vi "StartProgram.vi"() -> ()   [LabVIEW 2018]
uses:
  Type_Def/TypeDef_BMSData.ctl
  Type_Def/TypeDef_BmsStatus.ctl
  Type_Def/TypeDef_cRIOData.ctl
  Master/TypeDef_LoopPeriods.ctl
  <vilib>/Utility/error.llb/Error Cluster From Error Code.vi
  <vilib>/rvi/errors/niLvFpgaAdjustHostInterfaceError.vi
  <vilib>/rvi/interface/nirviReadWriteControl/nirviReadWriteControl.xnode
  <vilib>/NI_Real-Time Target Support.lvlib
  NiFpgaLv.dll
  <vilib>/rvi/interface/Simulation/niFpgaSimulationCallBeginRW.vi
panel:
  in  "error in (no error)":errorcluster
  out "FPGA VI Reference In 2":refnum<k20>
  in  "FPGA VI Reference In":refnum<k20>
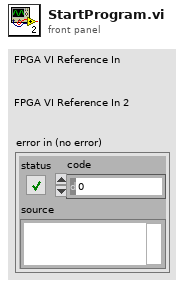
[diagram p1: front panel]
types:
  T1 = typedef "TypeDef_cRIOData.ctl" = cluster{"Time (ms)":dbl, "24V Battery (V)":dbl, "LowV Current (A)":dbl, "Fiducial Sensor (V)":dbl, "PV Pressure (psig)":dbl, "Flow Sensor (V)":dbl, "Temp Fairing (F)":dbl, "Temp Reservoir (F)":dbl, "HallEffect Right (in)":dbl, "HallEffect Left (in)":dbl, "PT Tank (psig)":dbl, "PT Clamp Right (psig)":dbl, "PT Clamp Left (psig)":dbl, "PT Brake (psig)":dbl, "PT Cooling (psig)":dbl, "Displacement (ft)":dbl, "Velocity (ft/s)":dbl}
  T2 = typedef "TypeDef_BMSData.ctl" = cluster{"Max Cell Voltage (V)":dbl, "Max Cell ID":dbl, "Min Cell Voltage (V)":dbl, "Min Cell ID":dbl, "State of Charge (%)":dbl, "Average Voltage (V)":dbl, "Voltage Delta (V)":dbl, "Pack Current (A)":dbl, "Pack Voltage (V)":dbl, "Max Resistance (Ohm)":dbl, "Min Resistance (Ohm)":dbl, "Average Resistance (Ohm)":dbl, "Delta Resistance (Ohm)":dbl, "Highest Temperature(F)":dbl, "BmsStatus":T3}
  T3 = typedef "TypeDef_BmsStatus.ctl" = cluster{"isFault":bool, "isolationMonitoring":bool}
  T4 = typedef "TypeDef_LoopPeriods.ctl" = cluster{"Control Period":i64, "DAQ Period":u32, "IMU Period":u32, "CAN Period":i64, "Nav Period":u32}
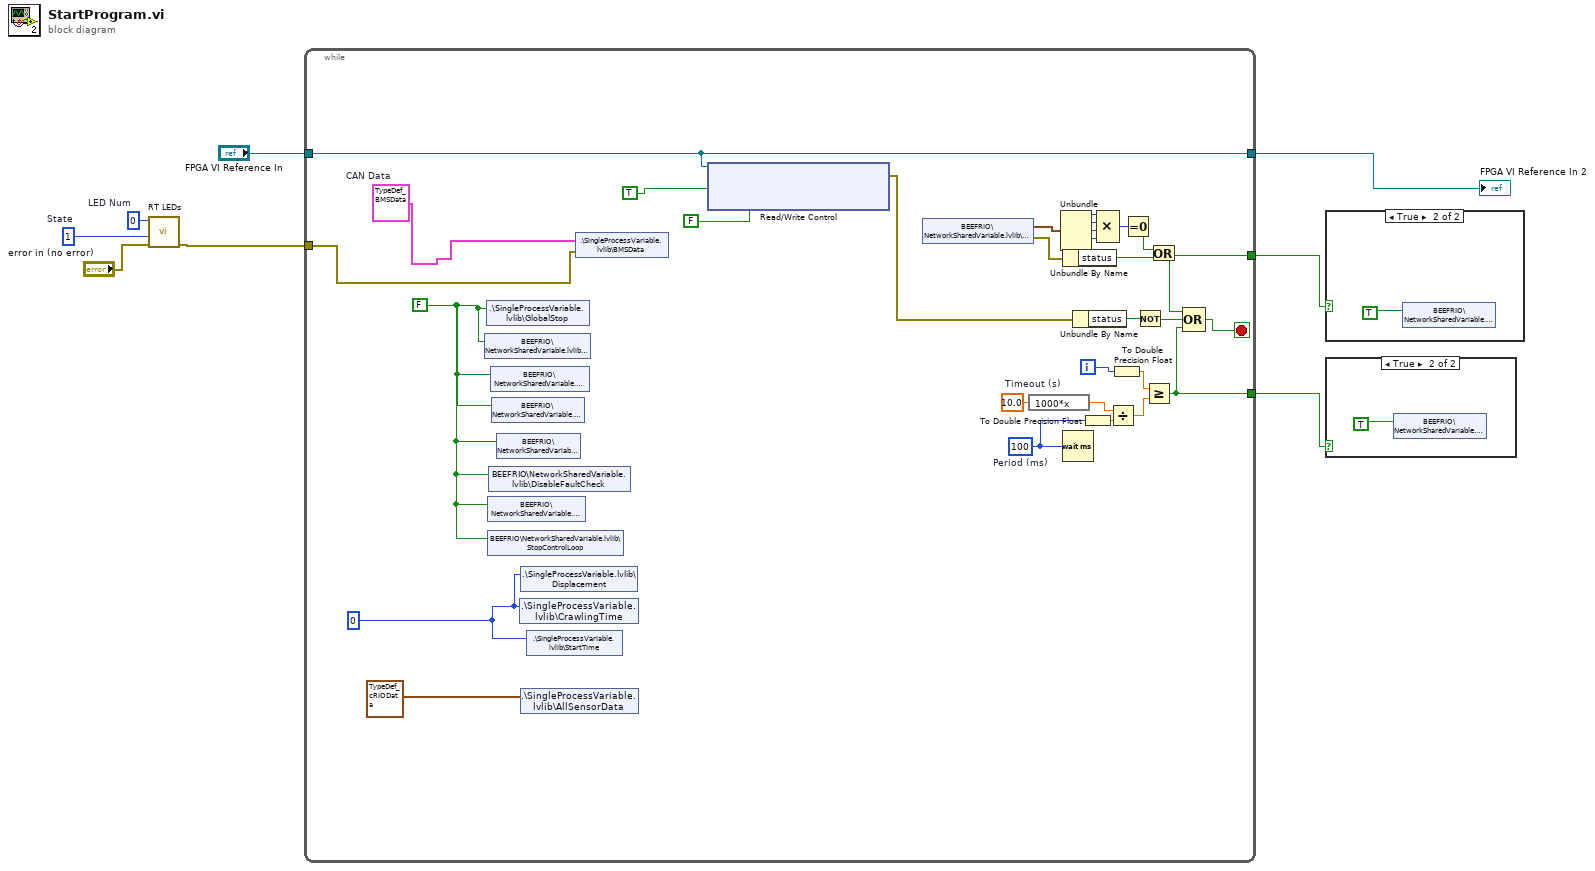
[diagram p0: block diagram]
diagram:
  w5 = 1  # State
  w6 = 0  # LED Num
  n1 = call <vilib>:"RT LEDs.vi"("error in (no error)"="error in (no error)", "State"=w5, "LED Num"=w6) -> ("error out"=w3:errorcluster)  [unwired: 3 in, 1 out]
  n2 = while {
    tunnel: [w32] -> w8
    tunnel: "FPGA VI Reference In" -> [w32]
    tunnel: w3 -> [w37]
    tunnel: [w12] -> w2
    tunnel: [w11] -> w1
    i -> [w9]
    stop <- w13 stop-if-true
    w29 = 10.0  # Timeout (s)
    w27 = u32 100  # Period (ms)
    w36 = i64 0 ("StartTime")
    w35 = FALSE ("GlobalStop")
    w38 = T2 {"Max Cell Voltage (V)"=0.0, "Max Cell ID"=0.0, "Min Cell Voltage (V)"=0.0, "Min Cell ID"=0.0, "State of Charge (%)"=0.0, "Average Voltage (V)"=0.0, "Voltage Delta (V)"=0.0, "Pack Current (A)"=0.0, "Pack Voltage (V)"=0.0, "Max Resistance (Ohm)"=0.0, "Min Resistance (Ohm)"=0.0, "Average Resistance (Ohm)"=0.0, "Delta Resistance (Ohm)"=0.0, "Highest Temperature(F)"=0.0, "BmsStatus"={"isFault"=FALSE, "isolationMonitoring"=FALSE}}  # CAN Data
    n3 = shared-variable "BEEFRIO\\NetworkSharedVariable.lvlib\\driveEnable"(w35) -> ()  [unwired: 1 in, 1 out]
    n4 = shared-variable ".\\SingleProcessVariable.lvlib\\GlobalStop"(w35) -> ()  [unwired: 1 in, 1 out]
    n5 = shared-variable "BEEFRIO\\NetworkSharedVariable.lvlib\\Precharge"(w35) -> ()  [unwired: 1 in, 1 out]
    n6 = shared-variable "BEEFRIO\\NetworkSharedVariable.lvlib\\StopControlLoop"(w35) -> ()  [unwired: 1 in, 1 out]
    n7 = shared-variable "BEEFRIO\\NetworkSharedVariable.lvlib\\DisableFaultCheck"(w35) -> ()  [unwired: 1 in, 1 out]
    n8 = shared-variable "BEEFRIO\\NetworkSharedVariable.lvlib\\Shutdown"(w35) -> ()  [unwired: 1 in, 1 out]
    n9 = shared-variable "BEEFRIO\\NetworkSharedVariable.lvlib\\ForceIdle"(w35) -> ()  [unwired: 1 in, 1 out]
    n10 = shared-variable "BEEFRIO\\NetworkSharedVariable.lvlib\\Launch"(w35) -> ()  [unwired: 1 in, 1 out]
    n11 = shared-variable ".\\SingleProcessVariable.lvlib\\CrawlingTime"(w36) -> ()  [unwired: 1 in, 1 out]
    n12 = shared-variable ".\\SingleProcessVariable.lvlib\\Displacement"(w36) -> ()  [unwired: 1 in, 1 out]
    n13 = shared-variable ".\\SingleProcessVariable.lvlib\\AllSensorData"(T1 {"Time (ms)"=0.0, "24V Battery (V)"=0.0, "LowV Current (A)"=0.0, "Fiducial Sensor (V)"=0.0, "PV Pressure (psig)"=0.0, "Flow Sensor (V)"=0.0, "Temp Fairing (F)"=0.0, "Temp Reservoir (F)"=0.0, "HallEffect Right (in)"=0.0, "HallEffect Left (in)"=0.0, "PT Tank (psig)"=0.0, "PT Clamp Right (psig)"=0.0, "PT Clamp Left (psig)"=0.0, "PT Brake (psig)"=0.0, "PT Cooling (psig)"=0.0, "Displacement (ft)"=0.0, "Velocity (ft/s)"=0.0} ("cRIO Data")) -> ()  [unwired: 1 in, 1 out]
    n14 = shared-variable ".\\SingleProcessVariable.lvlib\\StartTime"(w36) -> ()  [unwired: 1 in, 1 out]
    n15 = shared-variable ".\\SingleProcessVariable.lvlib\\BMSData"(w38, error in=w37) -> ()  [unwired: 1 out]
    n16 = xnode "Read/Write Control"("FPGA VI Reference In"=w32, "Enable RT Watchdog"=TRUE ("Boolean"), "RT Reset on Watchdog Failure?"=FALSE) -> ("error out"=w14:errorcluster)  [unwired: 1 in, 1 out]
    n17 = shared-variable "BEEFRIO\\NetworkSharedVariable.lvlib\\LoopPeriods"() -> (w23:T4, error out=w17:errorcluster)  [unwired: 1 in]
    n18 = expression code="1000*x"(w29) -> (w28:dbl)
    n19 = Unbundle(w23) -> ("Control Period"=w19:i64, "DAQ Period"=w21:u32, "IMU Period"=w20:u32, "CAN Period"=w22:i64)  [unwired: 1 out]
    n20 = Unbundle By Name(w17) -> ("status"=w15:bool)
    n21 = Wait (ms)(milliseconds to wait=w27) -> ()  [unwired: 1 out]
    n22 = Unbundle By Name(w14) -> ("status"=w31:bool)
    n23 = To Double Precision Float(number=w27) -> (double precision float=w25:dbl)
    n24 = Compound Arithmetic op=MULTIPLY(w19, w21, w20, w22) -> (w18:i64)
    n25 = Divide(x=w28, y=w25) -> (x/y=w26:dbl)
    n26 = To Double Precision Float(number=w9) -> (double precision float=w24:dbl)
    n27 = Equal To 0?(x=w18) -> (x = 0?=w16:bool)
    n28 = Not(x=w31) -> (.not. x?=w30:bool)
    n29 = Greater Or Equal?(x=w24, y=w26) -> (x >= y?=w11:bool)
    n30 = Or(x=w16, y=w15) -> (x .or. y?=w12:bool)
    n31 = Compound Arithmetic op=OR(w12, w30, w11) -> (w13:bool)
  }
  "FPGA VI Reference In 2" <- w8
  n32 = case shown="True" w2 {
    frame False {
    }
    frame True {
      n33 = shared-variable "BEEFRIO\\NetworkSharedVariable.lvlib\\ForceIdle"(TRUE ("Boolean")) -> ()  [unwired: 1 in, 1 out]
    }
  }
  n34 = case shown="True" w1 {
    frame False {
    }
    frame True {
      n35 = shared-variable "BEEFRIO\\NetworkSharedVariable.lvlib\\ForceIdle"(TRUE ("Boolean")) -> ()  [unwired: 1 in, 1 out]
    }
  }
